vi "config_read.vi"(7 "references":T1, 8 "error in (no error)":errorcluster) -> (0 "error out":errorcluster, 3 "configuration":T3)   [LabVIEW 2015, in "repub-dvr_nre.lvlib"]
doc: "This VI can be used to read the most recent configuration stored in the shared data notifier. It can be accessed publically and is vulnerable to read race conditions although the configuration should only change if the module is initialized or re-initialized."
uses:
  repub-dvr_nre.lvlib
  _controls/configuration.ctl
  private/_controls/input_command.ctl
  private/_controls/input.ctl
  private/_controls/output.ctl
  private/_controls/data.ctl
  _controls/references.ctl
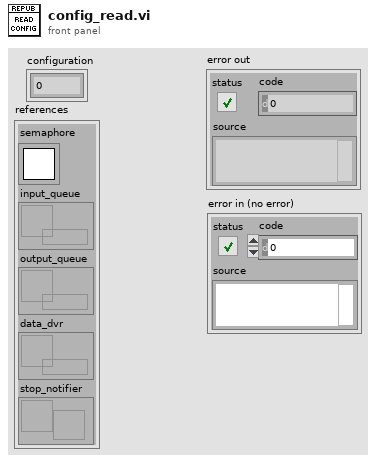
[diagram p1: front panel]
types:
  T1 = typedef "repub-dvr_nre.lvlib/references.ctl" = cluster{"semaphore":T2, "input_queue":refnum<queue>, "output_queue":refnum<queue>, "data_dvr":refnum<data-value>, "stop_notifier":refnum<notifier>}
  T2 = typedef "Semaphore RefNum" = refnum<k1>
  T3 = typedef "repub-dvr_nre.lvlib/configuration.ctl" = cluster{dbl}
  T4 = typedef "repub-dvr_nre.lvlib/data.ctl" = cluster{"configuration":T3, "working":cluster{"initialized":bool}}
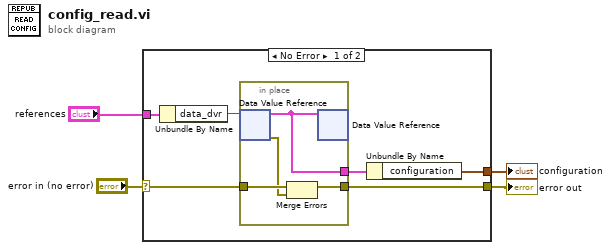
[diagram p0: block diagram]
diagram:
  n1 = case shown="No Error" "error in (no error)" {
    selector: "error in (no error)" -> [w7 w15]
    tunnel: [w6 w15] -> w3
    tunnel: [w10 _] -> w2
    tunnel: "references" -> [w9 _]
    frame No Error {
      n2 = Unbundle By Name(w9) -> ("data_dvr"=w8:refnum<data-value>)
      n3 = in-place {
        in-place-border: w7 -> [w14]
        in-place-border: [w12] -> w5
        in-place-border: [w11] -> w6
        n4 = in-place-dvr #1(w8) -> (w12:T4, w13:errorcluster)
        n5 = Merge Errors(w14, w13) -> (w11:errorcluster)
        n6 = in-place-dvr #1(w12) -> ()  [unwired: 2 out]
      }
      n7 = Unbundle By Name(w5) -> ("configuration"=w10:T3)
    }
    frame Error {
    }
  }
  "error out" <- w3
  "configuration" <- w2
